vi "SHUTDOWN.vi"(8 "error in (no error)":errorcluster, 11 "TecellaClient in":refnum<class "TecellaClient.lvclass">) -> (0 "error out":errorcluster, 3 "TecellaClient out":refnum<class "TecellaClient.lvclass">)   [LabVIEW 2009, in "TecellaClient.lvclass"]
uses:
  TecellaClient.lvclass
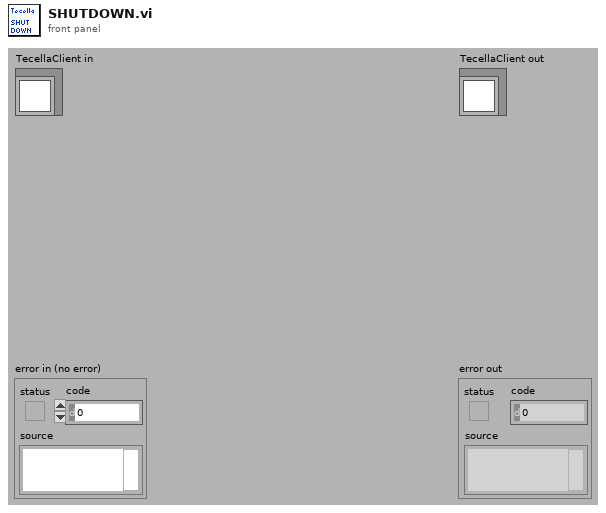
[diagram p1: front panel]
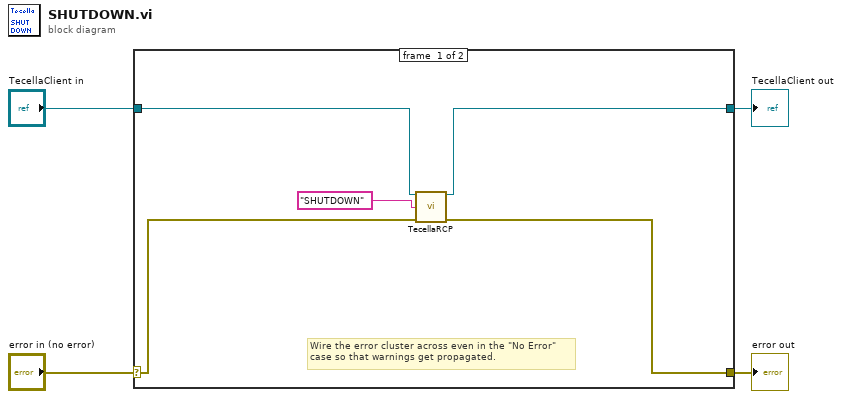
[diagram p0: block diagram]
diagram:
  n1 = case shown="No Error" "error in (no error)" {
    selector: "error in (no error)" -> [w7 w11]
    tunnel: [w6 w11] -> w3
    tunnel: [w8 w10] -> w1
    tunnel: "TecellaClient in" -> [w9 w10]
    frame #0 {
      # "Wire the error cluster across even in the \"No Error\"\ncase so that warnings get propagated."
      n2 = call-dynamic "TecellaRCP.vi"("TecellaClient in"=w9, "method"="SHUTDOWN" ("Name"), "error in (no error)"=w7) -> ("TecellaClient out"=w8:refnum<class "TecellaClient.lvclass">, "error out"=w6:errorcluster)  [unwired: 10 in, 1 out]
    }
    frame #1 {
    }
  }
  "error out" <- w3
  "TecellaClient out" <- w1
